vi "run path.vi"(8 "error in (no error)":errorcluster, 10 "Path Number":i32, 11 "CL57RS in":refnum<class "CL57RS.lvclass">) -> (0 "error out":errorcluster, 3 "CL57RS out":refnum<class "CL57RS.lvclass">)   [LabVIEW 2025, in "Motor.lvlib" / "CL57RS.lvclass"]
uses:
  CL57RS.lvclass
  CL57RS.lvclass/CL57RS.ctl
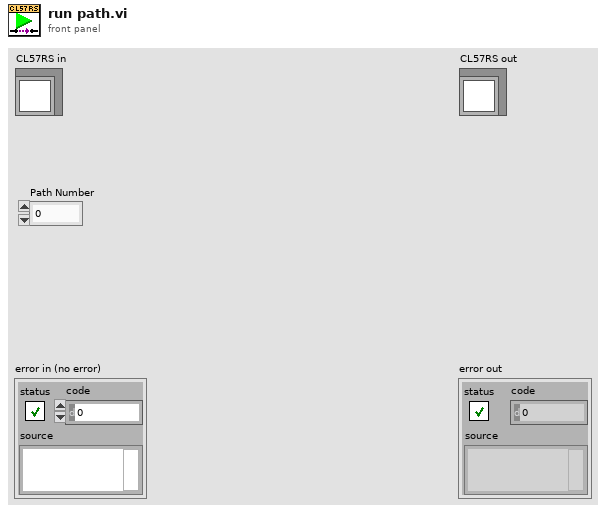
[diagram p1: front panel]
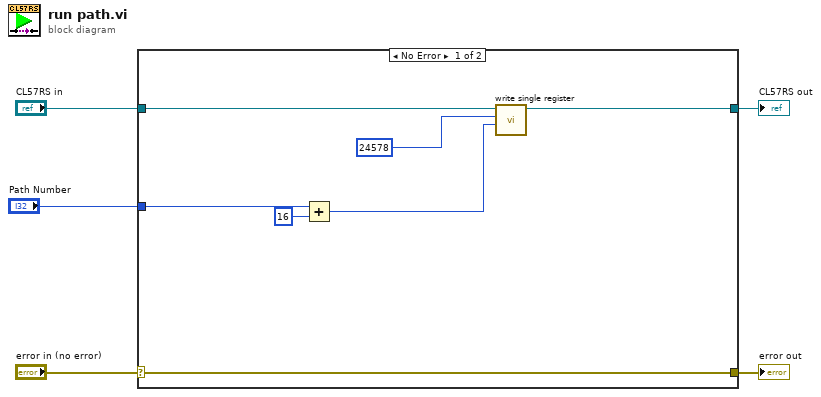
[diagram p0: block diagram]
diagram:
  n1 = case shown="No Error" "error in (no error)" {
    selector: "error in (no error)" -> [w12 w14]
    tunnel: [w12 w14] -> w4
    tunnel: [w8 w13] -> w2
    tunnel: "CL57RS in" -> [w7 w13]
    tunnel: "Path Number" -> [w6 _]
    frame No Error {
      n2 = Add(x=w6, y=16) -> (x+y=w9:i32)
      n3 = call "write single register.vi"("register to write"=w9, "address"=u16 24578, "CL57RS in"=w7) -> ("CL57RS out"=w8:refnum<class "CL57RS.lvclass">)  [unwired: 7 in, 1 out]
    }
    frame Error {
    }
  }
  "error out" <- w4
  "CL57RS out" <- w2
